vi "Read Lumps.vi"(8 "Error In":errorcluster, 10 "file (use dialog)":path, 11 "Cluster":T1) -> (0 "Error Out":errorcluster, 3 "Cluster 2":T1)   [LabVIEW 2017]
uses:
  WAD_MainCluster.ctl
  TextureList.ctl
  PatchList.ctl
  Lumps.ctl
  <vilib>/Utility/error.llb/Error Cluster From Error Code.vi
  <vilib>/Utility/error.llb/Search and Replace Pattern.vi
  <vilib>/ErrorRing/Error Ring.xnode
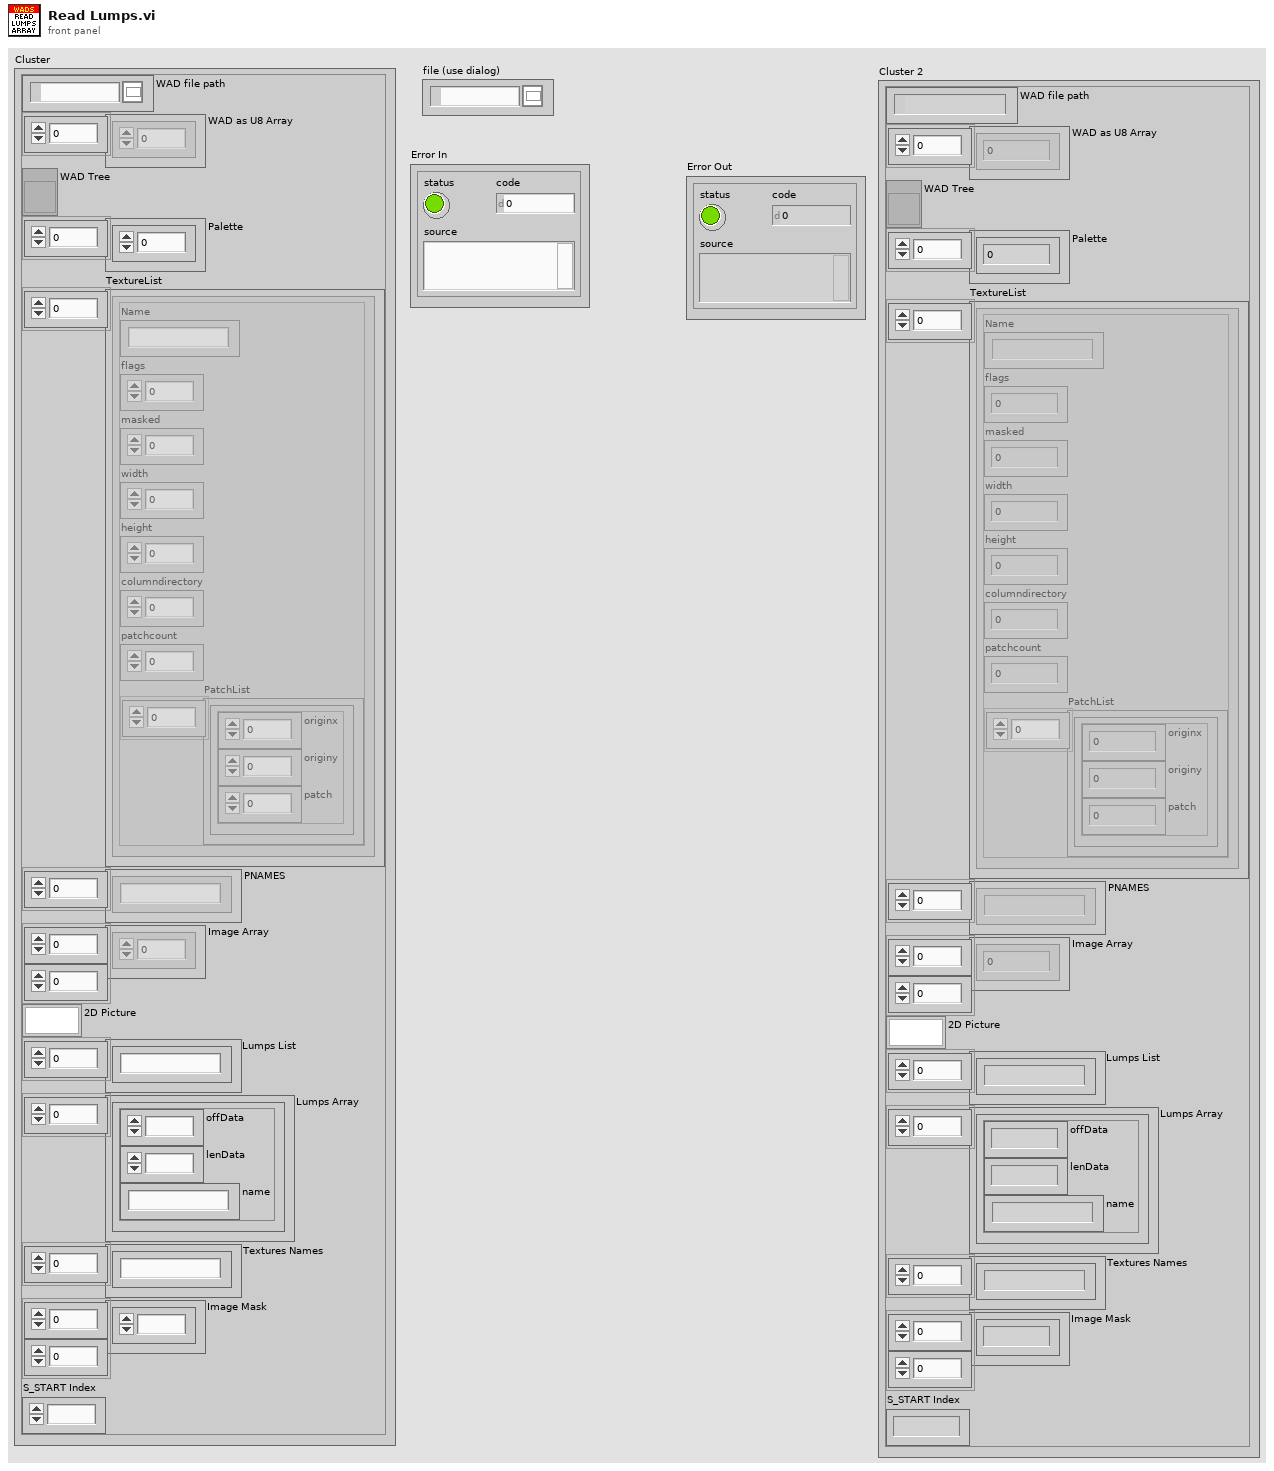
[diagram p1: front panel]
types:
  T1 = typedef "WAD_MainCluster.ctl" = cluster{"WAD file path":path, "WAD as U8 Array":u8[], "WAD Tree":refnum<vi>, "Palette":u32[], "TextureList":T2[], "PNAMES":string[], "Image Array":i16[][], "2D Picture":picture, "Lumps List":string[], "Lumps Array":T4[], "Textures Names":string[], "Image Mask":i16[][], "S_START Index":i32}
  T2 = typedef "TextureList.ctl" = cluster{"Name":string, "flags":u16, "masked":i16, "width":i16, "height":i16, "columndirectory":u32, "patchcount":i16, "PatchList":T3[]}
  T3 = typedef "PatchList.ctl" = cluster{"originx":i16, "originy":i16, "patch":i16}
  T4 = typedef "Lumps.ctl" = cluster{"offData":i32, "lenData":i32, "name":string}
  T5 = cluster{"Output I32":i32, "Output I32":i32, "String without \\00":string}
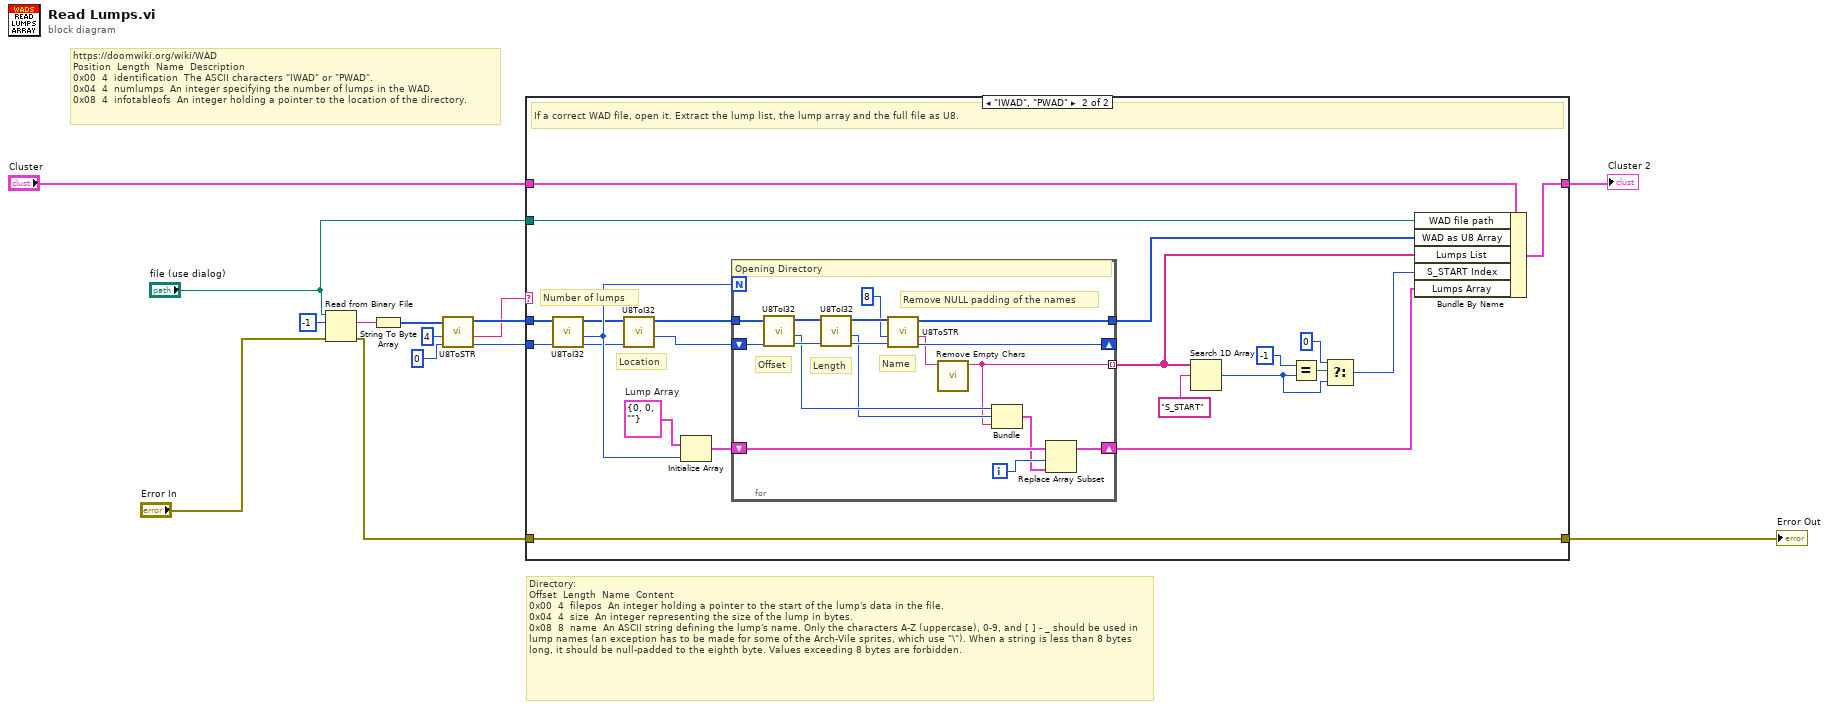
[diagram p0: block diagram]
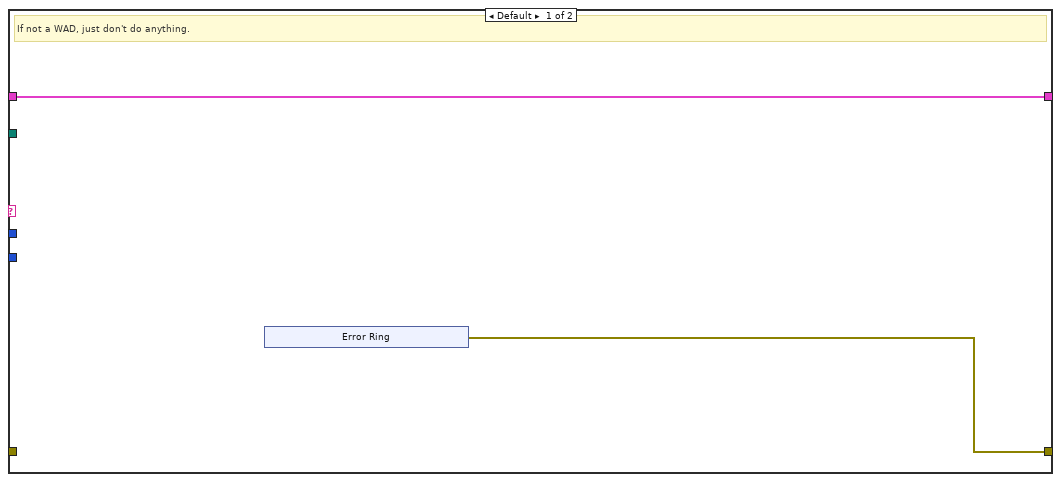
[diagram p2: hidden frame]
diagram:
  # "Directory:\nOffset \tLength \tName \tContent\n0x00 \t4 \tfilepos \tAn integer holding a pointer to the start of the lump's data in the file.\n0x04 \t4 \tsize \tAn integer representing the size of the lump in bytes.\n0x08 \t8 \tname \tAn ASCII string defining the lump's name. Only the characters A-Z (uppercase), 0-9, and [ ] - _ should be used in lump names (an exception has to be made for some of the Arch-Vile sprites, which use \"\\\"). When a string is less than 8 bytes long, it should be null-padded to the eighth byte. Values exceeding 8 bytes are forbidden."
  # "https://doomwiki.org/wiki/WAD\nPosition \tLength \tName \tDescription\n0x00 \t4 \tidentification \tThe ASCII characters \"IWAD\" or \"PWAD\".\n0x04 \t4 \tnumlumps \tAn integer specifying the number of lumps in the WAD.\n0x08 \t4 \tinfotableofs \tAn integer holding a pointer to the location of the directory."
  n1 = Read from Binary File(8:"Error In", 10:-1 ("count (1)"), 11:"file (use dialog)") -> (0:w5:errorcluster, 2:w11:string)  [unwired: 3 in, 2 out]
  n2 = String To Byte Array(string=w11) -> (unsigned byte array=w8:u8[])
  n3 = call "U8ToSTR.vi"("Index"=0 ("Count"), "Count"=4, "Input U8 Array"=w8) -> ("Index+Count"=w14:u32, "Output String"=w7:string, "Output U8 Array"=w13:u8[])  [unwired: 2 in]
  n4 = case shown="\"IWAD\", \"PWAD\"" w7 {
    tunnel: w14 -> [_ w36]
    tunnel: w13 -> [_ w35]
    tunnel: w5 -> [_ w34]
    tunnel: [w16 w34] -> w4
    tunnel: "Cluster" -> [w15 w33]
    tunnel: [w15 w30] -> w2
    tunnel: "file (use dialog)" -> [_ w32]
    frame Default {
      # "If not a WAD, just don't do anything."
      n5 = xnode "Error Ring"() -> ("error out"=w16:errorcluster)
    }
    frame "IWAD", "PWAD" {
      w40 = T4 {"offData"=0, "lenData"=0, "name"=""}  # Lump Array
      # "Number of lumps"
      # "Location"
      # "If a correct WAD file, open it. Extract the lump list, the lump array and the full file as U8."
      n6 = call "U8ToI32.vi"("Index"=w36, "Input U8 Array"=w35) -> ("Index+4"=w38:u32, "Output I32"=w41:i32, "Output U8 Array"=w37:u8[])  [unwired: 3 in]
      n7 = call "U8ToI32.vi"("Index"=w38, "Input U8 Array"=w37) -> ("Output I32"=w43:i32, "Output U8 Array"=w39:u8[])  [unwired: 3 in, 1 out]
      n8 = Initialize Array(w40, w41) -> (w42:T4[])
      n9 = for {
        N: w41 -> [_]
        tunnel: w39 -> [w60]
        shift-right: [w53] -> _
        shift-left: w43 -> [w59]
        tunnel: [w52] -> w31
        shift-right: [w49] -> w27
        shift-left: w42 -> [w51]
        tunnel: [w45] -> w28 mode=indexing
        i -> [w50]
        # "Remove NULL padding of the names"
        # "Name"
        # "Length"
        # "Offset"
        # "Opening Directory"
        n10 = call "U8ToI32.vi"("Index"=w59, "Input U8 Array"=w60) -> ("Index+4"=w57:u32, "Output I32"=w48:i32, "Output U8 Array"=w58:u8[])  [unwired: 3 in]
        n11 = call "U8ToI32.vi"("Index"=w57, "Input U8 Array"=w58) -> ("Index+4"=w55:u32, "Output I32"=w47:i32, "Output U8 Array"=w56:u8[])  [unwired: 3 in]
        n12 = call "U8ToSTR.vi"("Index"=w55, "Count"=8, "Input U8 Array"=w56) -> ("Index+Count"=w53:u32, "Output String"=w44:string, "Output U8 Array"=w52:u8[])  [unwired: 2 in]
        n13 = call "Remove Empty Chars.vi"("String with \\00"=w44) -> ("String without \\00"=w45:string)  [unwired: 10 in]
        n14 = Bundle("Output I32"=w48, "Output I32"=w47, "String without \\00"=w45) -> (w46:T5)  [unwired: 1 in]
        n15 = Replace Array Subset(array=w51, new element=w46, index=w50) -> (w49:T4[])
      }
      n16 = Search 1D Array(1D array=w28, element="S_START") -> (index of element=w23:i32)  [unwired: 1 in]
      n17 = Equal?(x=-1, y=w23) -> (x = y?=w25:bool)
      n18 = Select(t=0, s=w25, f=w23) -> (s? t:f=w22:i32)
      n19 = Bundle By Name(cluster=w33, "WAD file path"=w32, "WAD as U8 Array"=w31, "Lumps List"=w28, "S_START Index"=w22, "Lumps Array"=w27) -> (w30:T1)
    }
  }
  "Error Out" <- w4
  "Cluster 2" <- w2
